vi "controlword.vi"(8 "error in (no error)":errorcluster, 11 "controlword":T1(ring)) -> (0 "error out":errorcluster)   [LabVIEW 2014]
uses:
  <vilib>/CANopenLib/CANOPEN.llb/CANopen SDO Create.vi
  <vilib>/CANopenLib/CANOPEN.llb/CANopen SDO Write [U16].vi
  <vilib>/CANopenLib/CANOPEN.llb/CANopen SDO Close.vi
  <vilib>/CANopenLib/CANOPEN.llb/CANopen Interface Close.vi
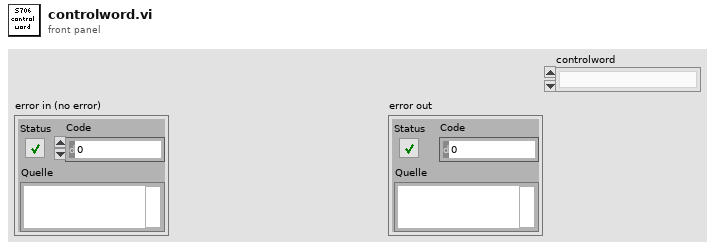
[diagram p1: front panel]
types:
  T1 = enum16{"", "Referenzfahrt start", "disable operation", "shut down", "enable operation", "quick stop", "disable voltage", "switch on"}
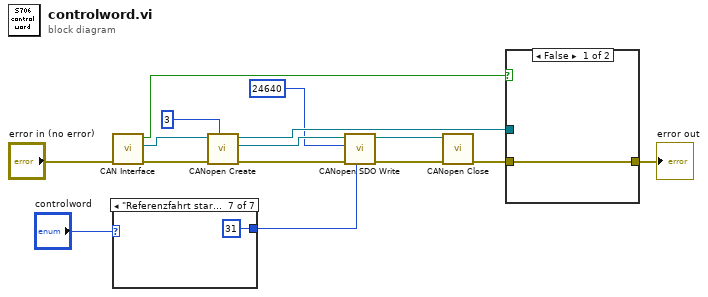
[diagram p0: block diagram]
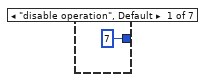
[diagram p2: hidden frame]
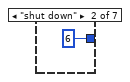
[diagram p3: hidden frame]
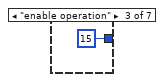
[diagram p4: hidden frame]
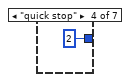
[diagram p5: hidden frame]
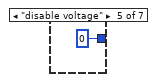
[diagram p6: hidden frame]
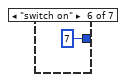
[diagram p7: hidden frame]
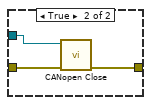
[diagram p8: hidden frame]
diagram:
  n1 = call "CAN Interface.vi"("error in (no error)"="error in (no error)") -> ("error out"=w10:errorcluster, "interface object out"=w11:refnum<k20>, "Interface schließen?"=w12:bool)  [unwired: 8 in]
  n2 = case shown="\"Referenzfahrt start\"" "controlword" {
    tunnel: [u16 7 ("U16 data") u16 6 ("U16 data") u16 15 ("U16 data") u16 2 ("U16 data") u16 0 ("U16 data") u16 7 ("U16 data") u16 31 ("U16 data")] -> w2
    frame "disable operation", Default {
    }
    frame "shut down" {
    }
    frame "enable operation" {
    }
    frame "quick stop" {
    }
    frame "disable voltage" {
    }
    frame "switch on" {
    }
    frame "Referenzfahrt start" {
    }
  }
  n3 = call-poly <vilib>:"CANopen Create.vi"("node-ID"=u8 3, "error in (no error)"=w10, "interface object in"=w11) -> ("error out"=w6:errorcluster, "SDO object out"=w8:refnum<k20>, "interface object out"=w7:refnum<k20>)  [unwired: 6 in]
  n4 = call-poly <vilib>:"CANopen SDO Write.vi"("U16 data"=w2, "error in (no error)"=w6, "object index"=u16 24640, "SDO object in"=w8) -> ("error out"=w5:errorcluster, "SDO object out"=w4:refnum<k20>)  [unwired: 5 in, 1 out]
  n5 = call-poly <vilib>:"CANopen Close.vi"("error in (no error)"=w5, "SDO object in"=w4) -> ("error out"=w14:errorcluster)  [unwired: 9 in]
  n6 = case shown="False" w12 {
    tunnel: w7 -> [_ w26]
    tunnel: w14 -> [w23 w25]
    tunnel: [w23 w24] -> w13
    frame False {
    }
    frame True {
      n7 = call-poly <vilib>:"CANopen Close.vi"("error in (no error)"=w25, "interface object in"=w26) -> ("error out"=w24:errorcluster)  [unwired: 9 in]
    }
  }
  "error out" <- w13
